vi "Read Sample Resistance.vi"(8 "error in (no error)":errorcluster, 10 "Action Data":variant, 11 "Controller in":refnum<class "Controller.lvclass">) -> (0 "error out":errorcluster, 3 "Controller out":refnum<class "Controller.lvclass">)   [LabVIEW 2020, in "Controller.lvlib" / "Controller.lvclass"]
uses:
  Controller.lvclass
  Actor_Scope/Actor_Scope/Scope_Action.ctl
  Controller.lvclass/Controller.ctl
  Actor_AFG/Actor_AFG Messages/AFG Config DC Voltage Msg/AFG Config DC Voltage Msg.lvclass/AFG Config DC Voltage Msg.ctl
  <vilib>/ActorFramework/Message Enqueuer/Message Enqueuer.lvclass/Message Enqueuer.ctl
  Actor_AFG/Actor_AFG Messages/AFG Setup Cycle Msg/AFG Setup Cycle Msg.lvclass/AFG Setup Cycle Msg.ctl
  Actor_AFG/Actor_AFG Messages/AFG Enable Output Msg/AFG Enable Output Msg.lvclass/AFG Enable Output Msg.ctl
  Actor_Scope/Actor_Scope Messages/Do Scope Action Msg/Do Scope Action Msg.lvclass/Do Scope Action Msg.ctl
  <vilib>/ActorFramework/Message Enqueuer/Enqueue.vi
  Actor_AFG/Actor_AFG Messages/AFG Config DC Voltage Msg/AFG Config DC Voltage Msg.lvclass
  C:/Program Files/National Instruments/LabVIEW 2020/vi.lib/ActorFramework/Message/Message.lvclass
  Actor_AFG/Actor_AFG Messages/AFG Setup Cycle Msg/AFG Setup Cycle Msg.lvclass
  Actor_AFG/Actor_AFG Messages/AFG Enable Output Msg/AFG Enable Output Msg.lvclass
  Actor_Scope/Actor_Scope Messages/Do Scope Action Msg/Do Scope Action Msg.lvclass
  Actor_NI6008/Actor_NI6008 Messages/NI6008 Enout Trigger Msg/NI6008 Enout Trigger Msg.lvclass
  <vilib>/ActorFramework/Message Priority Queue/Priority Enqueue.vi
  Actor_Scope/Actor_Scope/Actor_Scope.lvclass
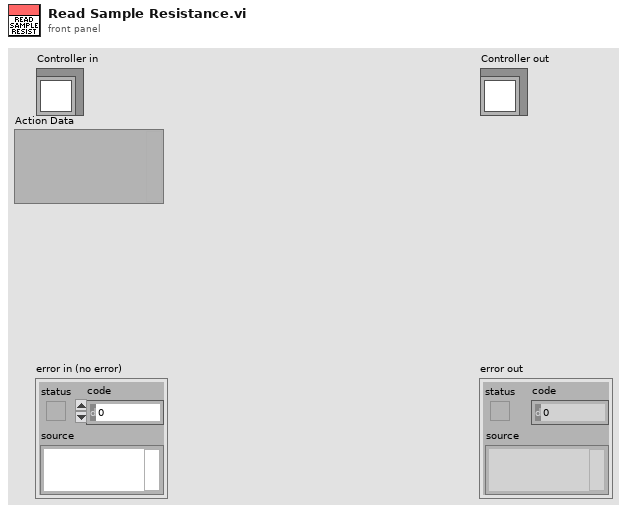
[diagram p1: front panel]
types:
  T1 = typedef "Actor_Scope.lvlib/Actor_Scope.lvclass/Scope_Action.ctl" = enum16{"Config Trigger", "Init Wfm Acq", "Read DC Res", "Read Wfm"}
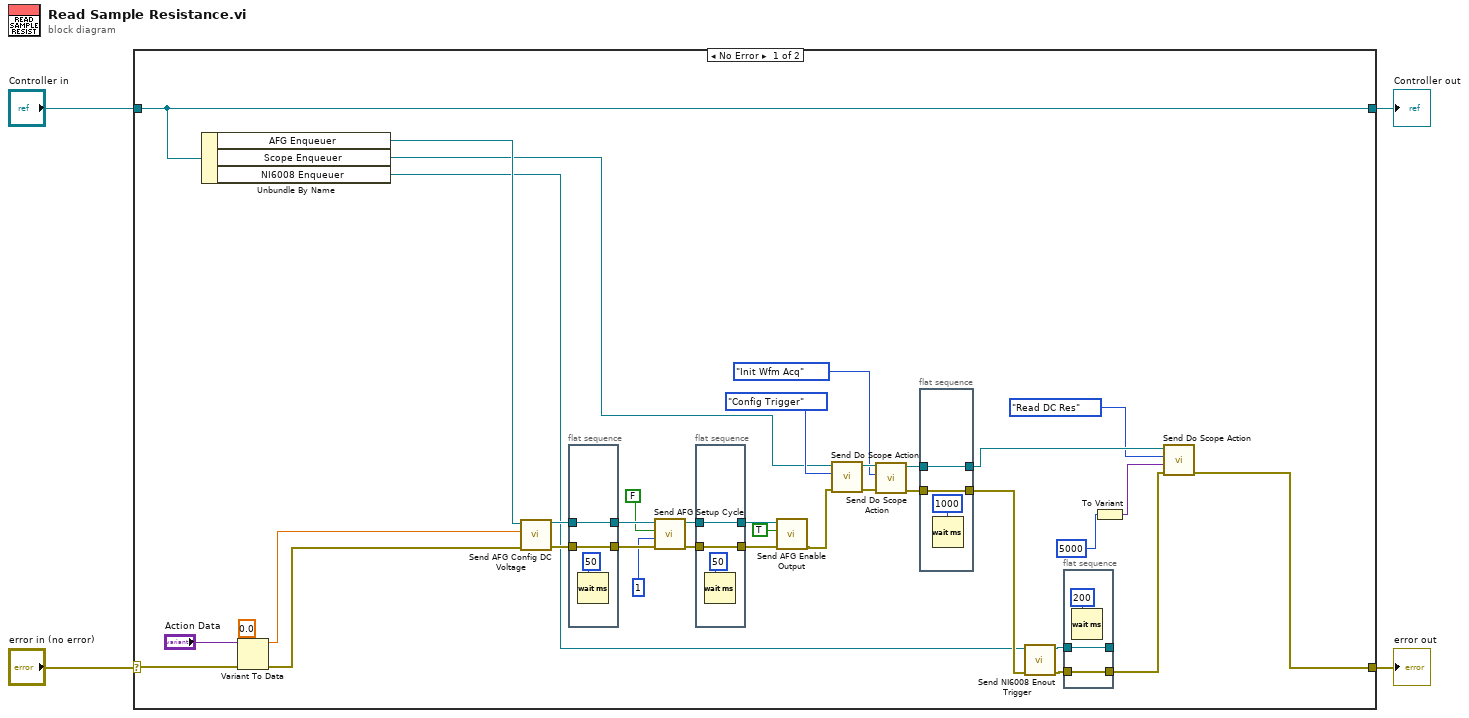
[diagram p0: block diagram]
diagram:
  n1 = case shown="No Error" "error in (no error)" {
    selector: "error in (no error)" -> [w37 w54]
    tunnel: [w5 w54] -> w3
    tunnel: [w40 w53] -> w1
    tunnel: "Controller in" -> [w40 w53]
    frame No Error {
      n2 = Unbundle By Name(w40) -> ("AFG Enqueuer"=w10:refnum<class "Message Enqueuer.lvclass">, "Scope Enqueuer"=w8:refnum<class "Message Enqueuer.lvclass">, "NI6008 Enqueuer"=w9:refnum<class "Message Enqueuer.lvclass">)
      n3 = Variant To Data(error in=w37, type=0.0, Variant="Action Data") -> (data=w7:dbl, error out=w6:errorcluster)
      n4 = call "Send AFG Config DC Voltage.vi"("error in (no error)"=w6, "DC Amplitude"=w7, "Message Enqueuer"=w10) -> ("error out"=w11:errorcluster, "Message Enqueuer out"=w12:refnum<class "Message Enqueuer.lvclass">)  [unwired: 7 in]
      n5 = flat-sequence {
        tunnel: w12 -> [w52]
        tunnel: [w52] -> w32
        tunnel: [w51] -> w31
        tunnel: w11 -> [w51]
        frame #0 {
          n6 = Wait (ms)(milliseconds to wait=u32 50) -> ()  [unwired: 1 out]
        }
      }
      n7 = call "Send AFG Setup Cycle.vi"("error in (no error)"=w31, "Cycles"=1 ("Cycle"), "Continuous"=FALSE ("Repeat"), "Message Enqueuer"=w32) -> ("error out"=w27:errorcluster, "Message Enqueuer out"=w28:refnum<class "Message Enqueuer.lvclass">)  [unwired: 6 in]
      n8 = flat-sequence {
        tunnel: w28 -> [w48]
        tunnel: w27 -> [w47]
        tunnel: [w48] -> w26
        tunnel: [w47] -> w16
        frame #0 {
          n9 = Wait (ms)(milliseconds to wait=u32 50) -> ()  [unwired: 1 out]
        }
      }
      n10 = call "Send AFG Enable Output.vi"("error in (no error)"=w16, "Enable Output (T: Enable)"=TRUE, "Message Enqueuer"=w26) -> ("error out"=w17:errorcluster)  [unwired: 7 in, 1 out]
      n11 = call "Send Do Scope Action.vi"("error in (no error)"=w17, "Scope Action"=Scope_Action."Config Trigger", "Message Enqueuer"=w8) -> ("error out"=w22:errorcluster, "Message Enqueuer out"=w23:refnum<class "Message Enqueuer.lvclass">)  [unwired: 7 in]
      n12 = call "Send Do Scope Action.vi"("error in (no error)"=w22, "Scope Action"=Scope_Action."Init Wfm Acq", "Message Enqueuer"=w23) -> ("error out"=w34:errorcluster, "Message Enqueuer out"=w33:refnum<class "Message Enqueuer.lvclass">)  [unwired: 7 in]
      n13 = flat-sequence {
        tunnel: w33 -> [w45]
        tunnel: w34 -> [w44]
        tunnel: [w45] -> w35
        tunnel: [w44] -> w15
        frame #0 {
          n14 = Wait (ms)(milliseconds to wait=u32 1000) -> ()  [unwired: 1 out]
        }
      }
      n15 = call "Send NI6008 Enout Trigger.vi"("error in (no error)"=w15, "Message Enqueuer"=w9) -> ("error out"=w13:errorcluster, "Message Enqueuer out"=w14:refnum<class "Message Enqueuer.lvclass">)  [unwired: 8 in]
      n16 = flat-sequence {
        tunnel: w14 -> [w42]
        tunnel: w13 -> [w41]
        tunnel: [w42] -> _
        tunnel: [w41] -> w36
        frame #0 {
          n17 = Wait (ms)(milliseconds to wait=u32 200) -> ()  [unwired: 1 out]
        }
      }
      n18 = To Variant(anything=5000 ("Time Out (ms)")) -> (Variant=w18:variant)
      n19 = call "Send Do Scope Action.vi"("error in (no error)"=w36, "Action Data In"=w18, "Scope Action"=Scope_Action."Read DC Res", "Message Enqueuer"=w35) -> ("error out"=w5:errorcluster)  [unwired: 6 in, 1 out]
    }
    frame Error {
    }
  }
  "error out" <- w3
  "Controller out" <- w1
